vi "RT FIFO Variables - target - networked.vi"   [LabVIEW 2017]
doc: "This example uses RT FIFO-enabled shared variables to publish data to remote machines without impacting determinism."
uses:
  <vilib>/Platform/TimedLoop/XDataNode/timing_clust.ctl
  <vilib>/Platform/TimedLoop/XDataNode/nitl_modes.ctl
  <vilib>/Platform/TimedLoop/XDataNode/wakeup.ctl
  <vilib>/platform/TimedLoop/XDataNode/XDataNode.xnode
  <vilib>/Platform/TimedLoop/XDataNode/XDNodeRunTimeDep.lvlib
panel:
  # "Overview: Uses RT FIFO-enabled shared variables to publish data to remote machines without impacting determinism.\nRequirements: LabVIEW Real-Time Module\nInstructions:\n1. In Measurement & Automation Explorer, ensure that LabVIEW Real-Time and the Network Variable Engine are installed on your RT target.\n2. From the Project Explorer window, set the IP address of your RT target.\n3. Run RT FIFO Variables - host - networked.vi.\n4. Run RT FIFO Variables - target - networked.vi.\n5. From the RT FIFO Variables - host - networked VI front panel, adjust the Amplitude slider, which will update the Result Data chart. \n6. Click the Stop button."
types:
  T1 = typedef "XDNodeRunTimeDep.lvlib/timing_clust.ctl" = cluster{"Expected End [f-1]":u64, "Actual End [f-1]":u64, "Finished Late? [f-1]":bool, "Expected End [i-1]":u64, "Actual End [i-1]":u64, "Finished Late? [i-1]":bool, "Expected Start [i]":u64, "Actual Start [i]":u64, "Expected Start [f]":u64, "Actual Start [f]":u64, "Source Name":string, "Structure Name":string, "Period":i64, "Deadline":i64, "Offset":i64, "Start":i64, "Priority":i32, "Timeout":i32, "Mode":T2, "Wakeup Reason":T3, "Error":errorcluster, "Source Type":string, "Secondary Source Type":string, "Global End Time":u64, "Global Start Time":u64, "Frame Duration":u64, "Iteration Duration":u64, "Assigned CPU":i32, "I/O Scan Engine Mode":u32}
  T2 = typedef "XDNodeRunTimeDep.lvlib/nitl_modes.ctl" = enum32{"No Change", "Process missed periods, maintain original phase", "Discard missed periods, maintain original phase", "Process missed periods, ignore original phase", "Discard missed periods, ignore original phase"}
  T3 = typedef "XDNodeRunTimeDep.lvlib/wakeup.ctl" = enum32{"Normal", "Aborted", "Asynchronous wakeup", "Timing source error", "Timed loop error", "Timeout"}
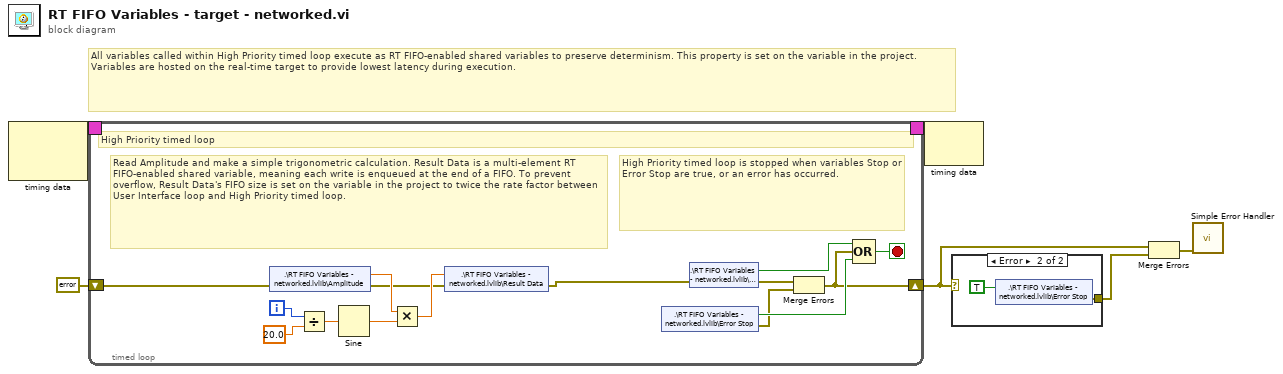
[diagram p0: block diagram]
diagram:
  # "All variables called within High Priority timed loop execute as RT FIFO-enabled shared variables to preserve determinism. This property is set on the variable in the project. Variables are hosted on the real-time target to provide lowest latency during execution."
  n1 = node-c288() -> (w6:T1)  [unwired: 1 in, 1 out]
  n2 = timed-loop "High Priority timed loop" {
    timing: w6 -> [_]
    timing-out: [_] -> w5
    shift-right: [w10] -> w2
    shift-left: errorcluster {"status"=FALSE, "code"=0, "source"=""} ("error in") -> [w14]
    i -> [w8]
    stop <- w21 stop-if-true
    # "Read Amplitude and make a simple trigonometric calculation. Result Data is a multi-element RT FIFO-enabled shared variable, meaning each write is enqueued at the end of a FIFO. To prevent overflow, Result Data's FIFO size is set on the variable in the project to twice the rate factor between User Interface loop and High Priority timed loop."
    # "High Priority timed loop is stopped when variables Stop or Error Stop are true, or an error has occurred."
    # "High Priority timed loop"
    n3 = shared-variable ".\\RT FIFO Variables - networked.lvlib\\Amplitude"(error in=w14) -> (w17:dbl, error out=w15:errorcluster)
    n4 = Divide(x=w8, y=20.0) -> (x/y=w7:dbl)
    n5 = Sine(x=w7) -> (sin(x)=w19:dbl)
    n6 = Multiply(x=w17, y=w19) -> (x*y=w16:dbl)
    n7 = shared-variable ".\\RT FIFO Variables - networked.lvlib\\Result Data"(w16, error in=w15) -> (error out=w13:errorcluster)
    n8 = shared-variable ".\\RT FIFO Variables - networked.lvlib\\Error Stop"() -> (w12:bool, error out=w9:errorcluster)  [unwired: 1 in]
    n9 = shared-variable ".\\RT FIFO Variables - networked.lvlib\\Stop"(error in=w13) -> (w18:bool, error out=w11:errorcluster)
    n10 = Merge Errors(w11, w9) -> (w10:errorcluster)
    n11 = Compound Arithmetic op=OR(w18, w10, w12) -> (w21:bool)
  }
  n12 = node-c288(w5) -> ()  [unwired: 1 out]
  n13 = case shown="Error" w2 {
    tunnel: [_ w24] -> w3
    frame No Error {
    }
    frame Error {
      n14 = shared-variable ".\\RT FIFO Variables - networked.lvlib\\Error Stop"(TRUE ("Error Stop")) -> (error out=w24:errorcluster)  [unwired: 1 in]
    }
  }
  n15 = Merge Errors(w2, w3) -> (w4:errorcluster)
  n16 = call <vilib>:"Simple Error Handler.vi"("error in (no error)"=w4) -> ()  [unwired: 4 in, 5 out]
